vi "Read RunTimeObjectType.vi"(8 "error in (no error)":errorcluster, 11 "RunTimeObjectsSection in":refnum<class "RunTimeObjectsSection.lvclass">) -> (0 "error out":errorcluster, 2 "RunTimeObjectType":T1, 3 "RunTimeObjectsSection out":refnum<class "RunTimeObjectsSection.lvclass">)   [LabVIEW 2019, in "RunTimeObjectsSection.lvclass"]
uses:
  RunTimeObjectsSection.lvclass
  Controls/RunTimeObjectTypes.ctl
  RunTimeObjectsSection.lvclass/RunTimeObjectsSection.ctl
  Configuration Tool.lvlib
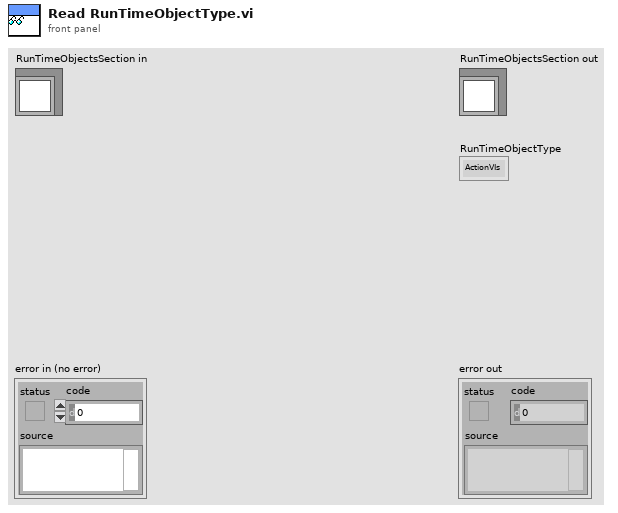
[diagram p1: front panel]
types:
  T1 = typedef "Configuration Tool.lvlib/RunTimeObjectTypes.ctl" = enum16{"ActionVIs", "ButtonList", "RunTimeMenu"}
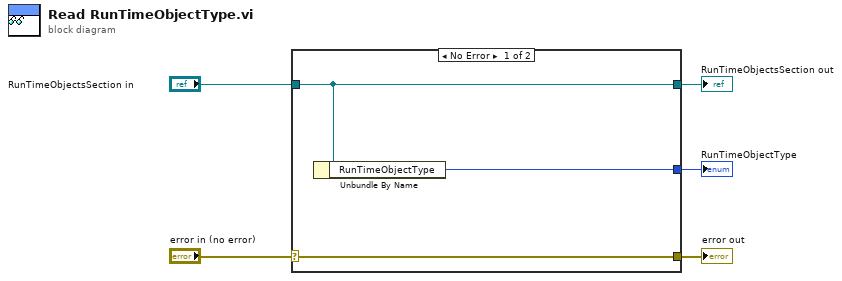
[diagram p0: block diagram]
diagram:
  n1 = case shown="No Error" "error in (no error)" {
    selector: "error in (no error)" -> [w8 w9]
    tunnel: [w8 w9] -> w4
    tunnel: [w7 w10] -> w2
    tunnel: "RunTimeObjectsSection in" -> [w7 w10]
    tunnel: [w6 _] -> w1
    frame No Error {
      n2 = Unbundle By Name(w7) -> ("RunTimeObjectType"=w6:T1)
    }
    frame Error {
    }
  }
  "error out" <- w4
  "RunTimeObjectsSection out" <- w2
  "RunTimeObjectType" <- w1
